vi "HW_Setup_3.vi"(0 "VISA resource name in":refnum<visa-resource-name>="Tracker", 5 "Acquisition FPS":T2, 9 "Close port? (F)":bool, 11 "error in":errorcluster) -> (3 "FPS status":i32=80, 4 "VISA resource name out":refnum<visa-resource-name>, 6 "HW information":string, 8 "SB type (size)":T1, 10 "Sync capability":u8, 14 "Instrument OK?":bool, 15 "error out":errorcluster)   [LabVIEW 2018, in "HW Interaction.lvlib"]
uses:
  HW Interaction.lvlib
  SubVi's/Controls/CTL_Acquisition_speed_selector.ctl
  Public API/Typedefs/CTL_Sensor_board_type_(size).ctl
  Common_Resources.lvlib
panel:
  out "Sensor board size":string
  out "Sync mode status":string
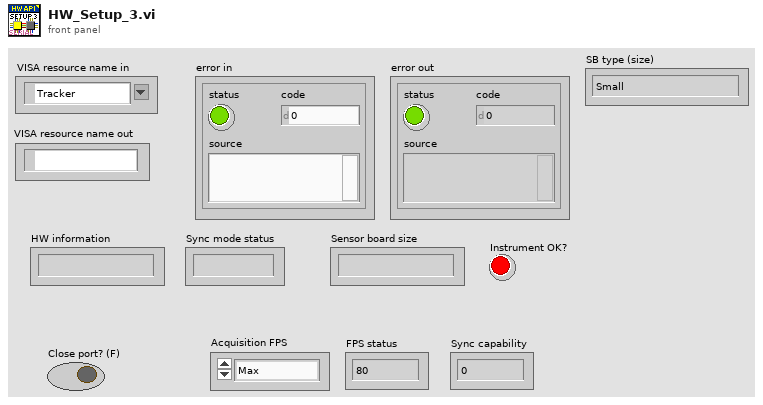
[diagram p1: front panel]
types:
  T1 = typedef "HW Interaction.lvlib/CTL_Sensor_board_type_(size).ctl" = enum16{"Small", "Large"}
  T2 = typedef "Common_Resources.lvlib/CTL_Acquisition_speed_selector.ctl" = enum16{"Max", "Optimal", "Eco"}
  T3 = typedef "HW Interaction.lvlib/CTL_HW_Init_outcome.ctl" = cluster{"VISA resource name":refnum<visa-resource-name>, "FW version information":string, "Sensor board size":string, "Sync mode status":string, "FPS status":i32, "Instrument OK?":bool}
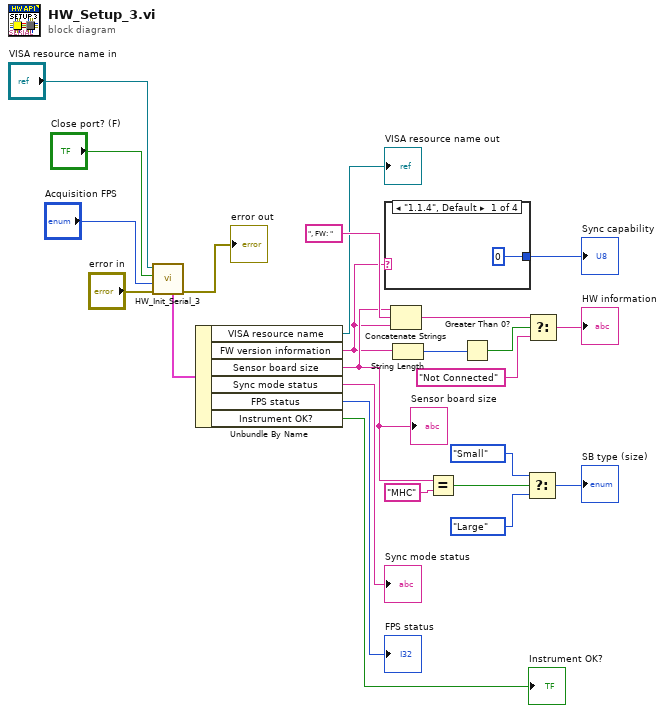
[diagram p0: block diagram]
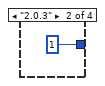
[diagram p2: hidden frame]
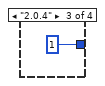
[diagram p3: hidden frame]
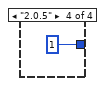
[diagram p4: hidden frame]
diagram:
  n1 = call "HW_Init_Serial_3.vi"("error in"="error in", "Acquisition FPS"="Acquisition FPS", "Close port? (F)"="Close port? (F)", "VISA resource name"="VISA resource name in") -> ("error out"=→"error out":errorcluster, "Init status"=w1:T3)  [unwired: 3 in, 3 out]
  n2 = Unbundle By Name(w1) -> ("VISA resource name"=→"VISA resource name out":refnum<visa-resource-name>, "FW version information"=w4:string, "Sensor board size"=w9:string, "Sync mode status"=→"Sync mode status":string, "FPS status"=→"FPS status":i32, "Instrument OK?"=→"Instrument OK?":bool)
  "Sensor board size" <- w9
  n3 = case shown="\"1.1.4\", Default" w4 {
    tunnel: [u8 0 u8 1 u8 1 u8 1] -> w13
    frame "1.1.4", Default {
    }
    frame "2.0.3" {
    }
    frame "2.0.4" {
    }
    frame "2.0.5" {
    }
  }
  "Sync capability" <- w13
  n4 = Concatenate Strings(w9, ", FW: " ("string"), w4) -> (w17:string)
  n5 = String Length(string=w4) -> (length=w15:i32)
  n6 = Equal?(x=w9, y="MHC") -> (x = y?=w11:bool)
  n7 = Greater Than 0?(x=w15) -> (x > 0?=w18:bool)
  n8 = Select(t=CTL_Sensor_board_type_(size)."Small" ("Sensor board type"), s=w11, f=CTL_Sensor_board_type_(size)."Large" ("Sensor board type")) -> (s? t:f=→"SB type (size)":T1)
  n9 = Select(t=w17, s=w18, f="Not Connected") -> (s? t:f=→"HW information":string)
